vi "view.vi"() -> ()   [LabVIEW 2022 SP3]
panel:
  in  "File Path":path
  in  "Save File Path":path
  out "Image":T1(plugin-control)
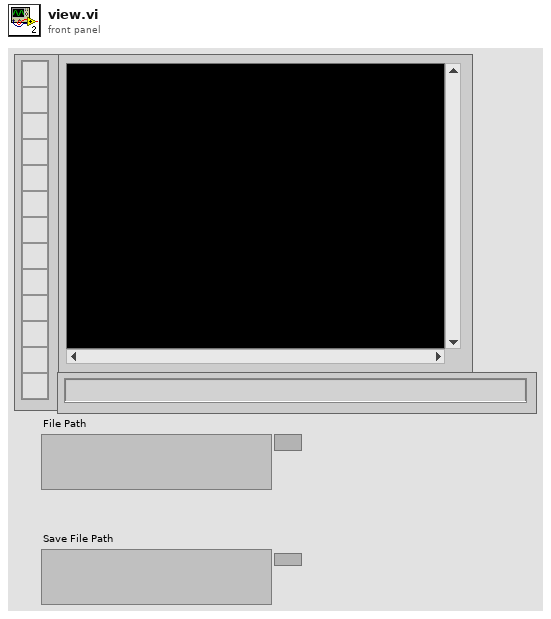
[diagram p1: front panel]
types:
  T1 = typedef "IMAQ Image.ctl" = refnum<image>
  T2 = cluster{"Desired Font (Application)":enum16{"User-specified Font", "Application Font", "System Font", "Dialog Font"}, "[User-specified Font]":cluster{"Font Name":string, "Size":i16, "Strikeout?":bool, "Italic?":bool, "Underline?":bool, "Outline?":bool, "Shadow?":bool, "Bold?":bool, "Rotation Angle":dbl}, "Horizontal Alignment":i16, "Vertical Alignment":i16}
  T3 = typedef "Image Type" = u32
  T4 = cluster{"Global Rectangle":i32[], "Contours":cluster{"Contour Type":u32, "ROI Type":u32, "Points":i32[]}[]}
  T5 = cluster{"Contour Type":u32, "ROI Type":u32, "Points":i32[]}[]
  T6 = cluster{"Contour Type":u32, "ROI Type":u32, "Points":i32[]}
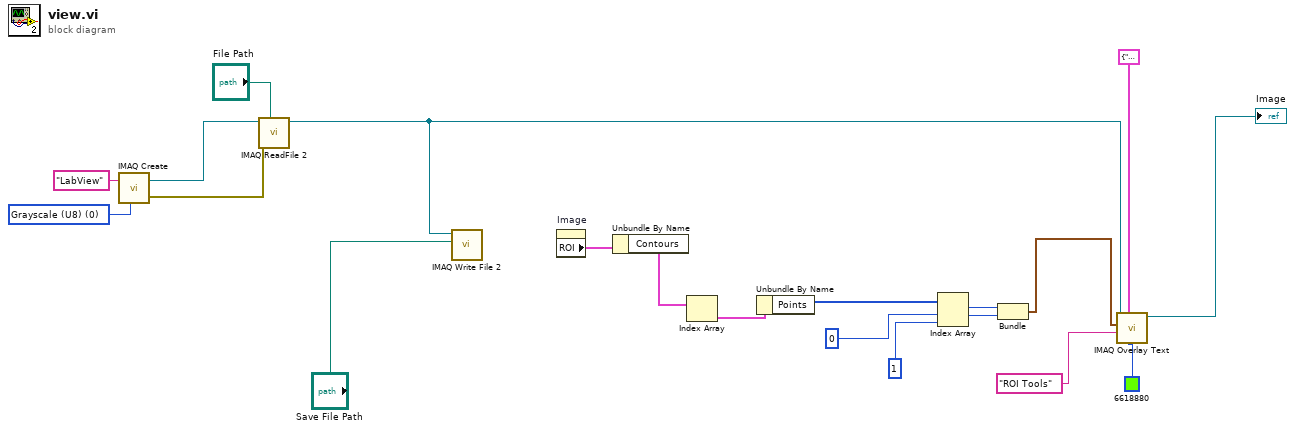
[diagram p0: block diagram]
diagram:
  w17 = T3 0 items=["Grayscale (U8)", "Grayscale (I16)", "Grayscale (SGL)", "Complex (CSG)", "RGB (U32)", "HSL (U32)", "RGB (U64)", "Grayscale (U16)"] ("Image Type")
  n1 = call "IMAQ Create"("Image Name"="LabView", "Image Type"=w17) -> ("New Image"=w20:T1, "error out"=w19:errorcluster)  [unwired: 3 in]
  n2 = call "IMAQ ReadFile 2"("File Path"="File Path", "error in (no error)"=w19, "Image"=w20) -> ("Image Out"=w4:T1)  [unwired: 4 in, 4 out]
  n3 = call-poly "IMAQ Write File 2"("File Path"="Save File Path", "Image"=w4) -> ()  [unwired: 8 in, 2 out]
  n4 = property on="Image" class="ImageControl"() -> ("ROI"=w14:T4)  [unwired: 2 in, 2 out]
  n5 = Unbundle By Name(w14) -> ("Contours"=w13:T5)
  n6 = Index Array(array=w13) -> (element=w12:T6)  [unwired: 1 in]
  n7 = Unbundle By Name(w12) -> ("Points"=w11:i32[])
  n8 = Index Array(array=w11, index #1=0 ("索引"), index #2=1 ("索引")) -> (element #1=w8:i32, element #2=w7:i32)
  n9 = Bundle(w8, w7) -> (w6:cluster{i32, i32})  [unwired: 1 in]
  n10 = call "IMAQ Overlay Text"("Text Color (black)"=u32 6618880, "Font, Size & Style"=T2 {"Desired Font (Application)"=enum."Application Font", "[User-specified Font]"={"Font Name"="", "Size"=40, "Strikeout?"=FALSE, "Italic?"=FALSE, "Underline?"=FALSE, "Outline?"=FALSE, "Shadow?"=FALSE, "Bold?"=FALSE, "Rotation Angle"=0.0}, "Horizontal Alignment"=0, "Vertical Alignment"=0}, "String"="ROI Tools", "Origin"=w6, "Image"=w4) -> ("Image Out"=→"Image":T1)  [unwired: 5 in, 1 out]
